vi "Untitled 1.vi"() -> ()   [LabVIEW 2020]
panel:
  out "AI1":dbl
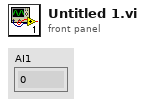
[diagram p1: front panel]
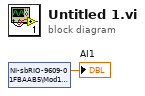
[diagram p0: block diagram]
diagram:
  n1 = shared-variable "NI-sbRIO-9609-01FBAAB5\\Mod1\\AI1"() -> (→"AI1":dbl)  [unwired: 1 in, 1 out]
